vi "Create All Message Queues.vi"(8 "error in (no error)":errorcluster) -> (0 "error out":errorcluster, 3 "Message Queues out":T1)   [LabVIEW 2017, in "ImageAcquisitionLibrary.lvlib" / "MessageQueue.lvlib"]
doc: "This VI creates and initializes all the message queues for your application. If your application requires more than one message queue, right-click the \"Message Queues\" constant above and select Open Type Def. Add the new Message Queue(s) to the type definition, then initialize them in this VI."
uses:
  MessageQueue.lvlib
  All Message Queues.ctl
  Message Cluster.ctl
  Enqueue Message (Single).vi
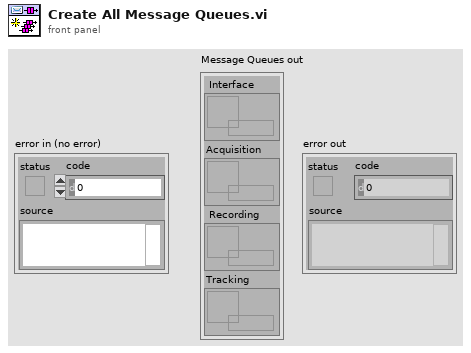
[diagram p1: front panel]
types:
  T1 = typedef "ImageAcquisitionLibrary.lvlib/MessageQueue.lvlib/All Message Queues.ctl" = cluster{" Interface":refnum<queue>, "Acquisition":refnum<queue>, " Recording":refnum<queue>, "Tracking":refnum<queue>}
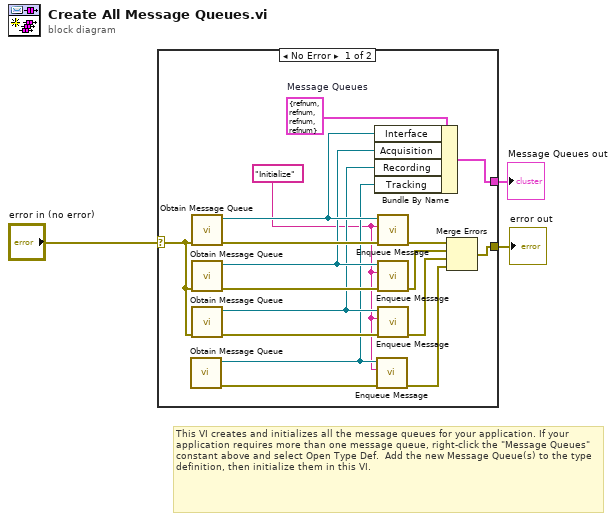
[diagram p0: block diagram]
diagram:
  # "This VI creates and initializes all the message queues for your application. If your application requires more than one message queue, right-click the \"Message Queues\" constant above and select Open Type Def.  Add the new Message Queue(s) to the type definition, then initialize them in this VI."
  n1 = case shown="No Error" "error in (no error)" {
    selector: "error in (no error)" -> [w10 w21]
    tunnel: [w16 w21] -> w3
    tunnel: [w19 _] -> w2
    frame No Error {
      w4 = "Initialize" ("Message")
      w20 = T1 {" Interface"=refnum, "Acquisition"=refnum, " Recording"=refnum, "Tracking"=refnum}  # Message Queues
      n2 = call "Obtain Message Queue.vi"() -> ("error out"=w7:errorcluster, "Message Queue"=w5:refnum<queue>)  [unwired: 10 in]
      n3 = call "Obtain Message Queue.vi"("error in (no error)"=w10) -> ("error out"=w18:errorcluster, "Message Queue"=w15:refnum<queue>)  [unwired: 9 in]
      n4 = call "Obtain Message Queue.vi"("error in (no error)"=w10) -> ("error out"=w12:errorcluster, "Message Queue"=w9:refnum<queue>)  [unwired: 9 in]
      n5 = call "Obtain Message Queue.vi"("error in (no error)"=w10) -> ("error out"=w11:errorcluster, "Message Queue"=w8:refnum<queue>)  [unwired: 9 in]
      n6 = Bundle By Name(cluster=w20, "Interface"=w15, "Acquisition"=w9, "Recording"=w8, "Tracking"=w5) -> (w19:T1)
      n7 = call-poly "Enqueue Message.vi"("error in (no error)"=w7, "Message"=w4, "Message Queue"=w5) -> ("error out"=w6:errorcluster)  [unwired: 7 in, 1 out]
      n8 = call-poly "Enqueue Message.vi"("error in (no error)"=w18, "Message"=w4, "Message Queue"=w15) -> ("error out"=w17:errorcluster)  [unwired: 7 in, 1 out]
      n9 = call-poly "Enqueue Message.vi"("error in (no error)"=w12, "Message"=w4, "Message Queue"=w9) -> ("error out"=w14:errorcluster)  [unwired: 7 in, 1 out]
      n10 = call-poly "Enqueue Message.vi"("error in (no error)"=w11, "Message"=w4, "Message Queue"=w8) -> ("error out"=w13:errorcluster)  [unwired: 7 in, 1 out]
      n11 = Merge Errors(w17, w14, w13, w6) -> (w16:errorcluster)
    }
    frame Error {
    }
  }
  "Message Queues out" <- w2
  "error out" <- w3
